vi "Go Home Sub_VI.vi"(8 "error in (no error)":errorcluster, 9 "stop":bool, 10 "Homing Freq":dbl format="%#_13g", 11 "Homing Duty %":dbl format="%#_13g") -> (0 "error out":errorcluster, 2 "Motor Status out":T2 {"Homing Duty %" format="%#_13g"; "Homing Freq" format="%#_13g"})   [LabVIEW 2017]
uses:
  X-Y Manipulator go home/Go Home State type def.ctl
panel:
  out "Y Velocity (mm/s)":dbl format="%#_3g"
  out "Y-axis distance":dbl
  out "X Velocity (mm/s)":dbl format="%#_3g"
  out "X-axis distance":dbl
  out "Y Axis State":T1
  out "X Axis state":T1
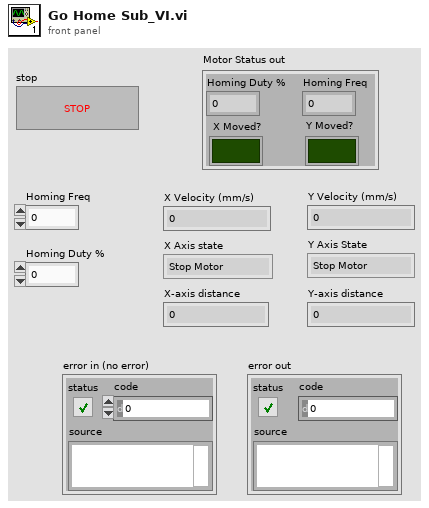
[diagram p1: front panel]
types:
  T1 = typedef "Go Home State type def.ctl" = enum16{"Stop Motor", "Read Input", "Drive Motor"}
  T2 = cluster{"Homing Freq":dbl, "Homing Duty %":dbl, "X Moved?":bool, "Y Moved?":bool}
  T3 = typedef "Encoder Count Direction Enum.ctl" = enum16{"Counting Up", "Counting Down"}
  T4 = cluster{"Y-axis rev count":dbl, "Y-axis distance":dbl, "X-axis rev count":dbl, "X-axis distance":dbl, "Y-axis direction":T3, "X-axis direction":T3, "X-counter val":i32, "Y-counter val":i32, "Reset X":bool, "Reset Y":bool}
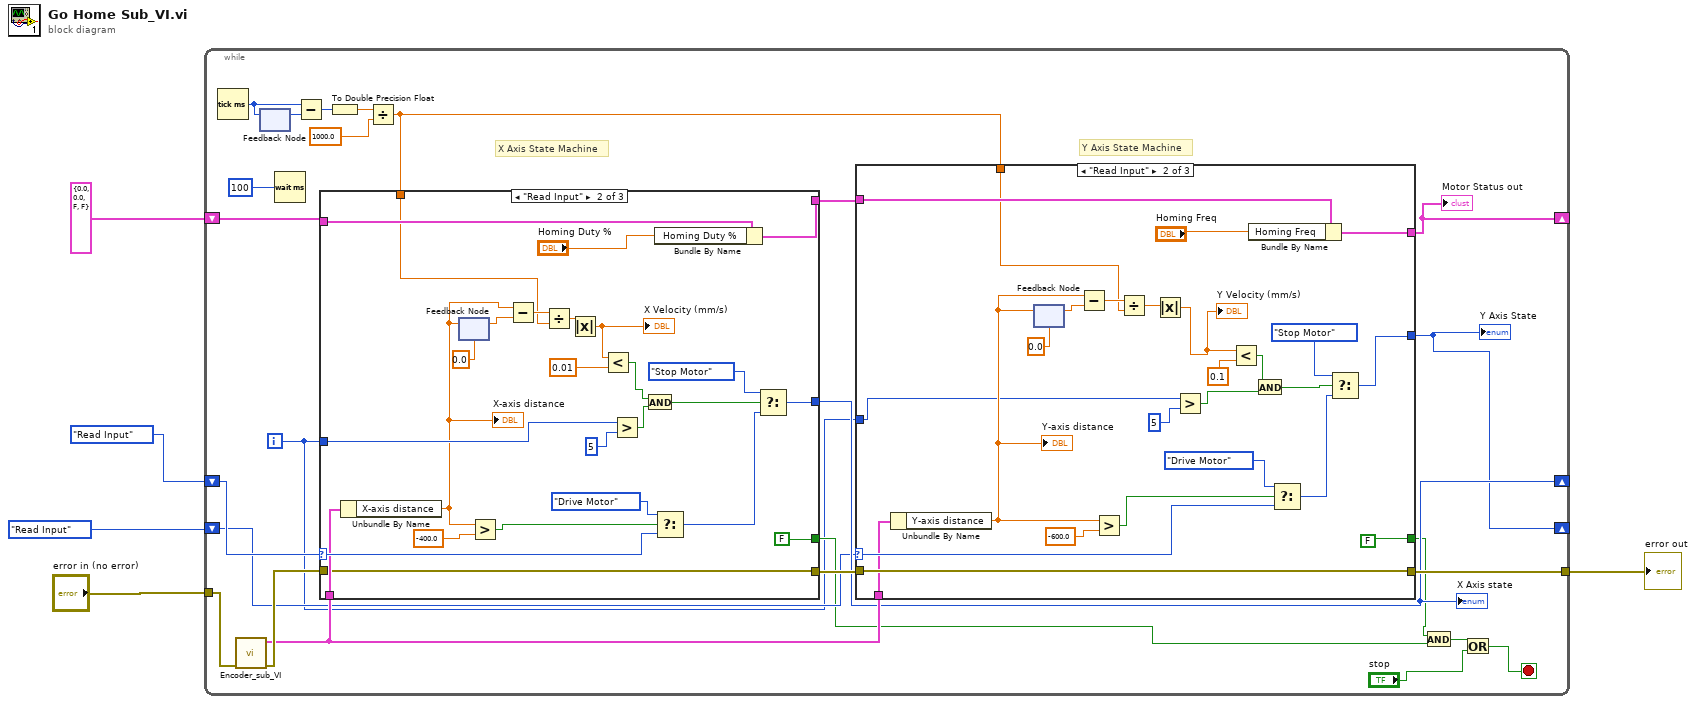
[diagram p0: block diagram]
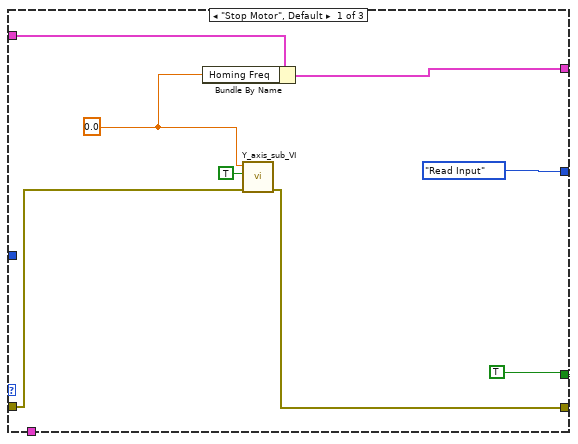
[diagram p2: hidden frame]
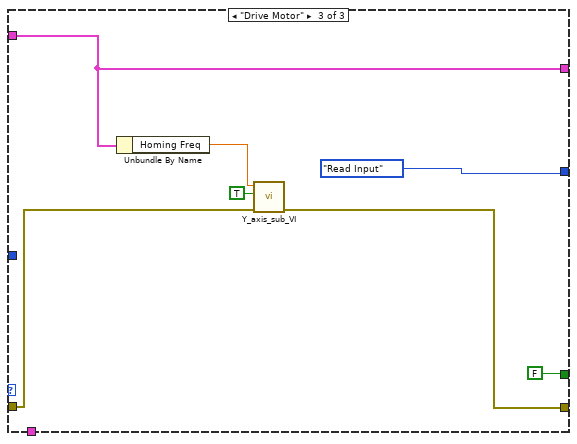
[diagram p3: hidden frame]
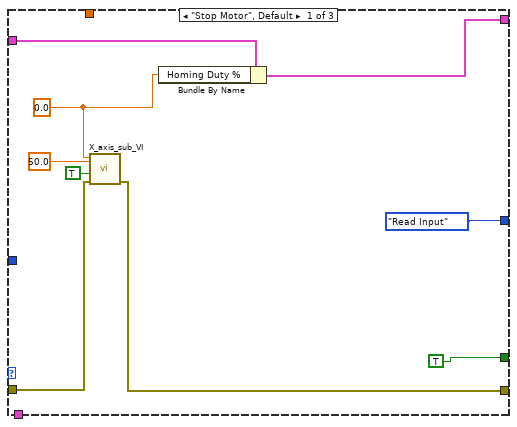
[diagram p4: hidden frame]
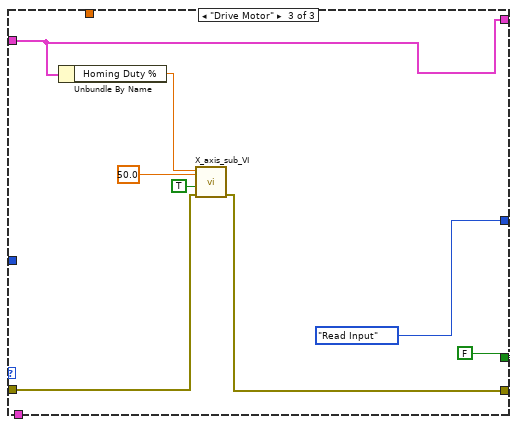
[diagram p5: hidden frame]
diagram:
  n1 = while {
    tunnel: "error in (no error)" -> [w29]
    tunnel: [w25] -> w2
    shift-right: [w21] -> _
    shift-left: Go_Home_State_type_def."Read Input" ("Enum 2") -> [w28]
    shift-right: [w26] -> _
    shift-left: T2 {"Homing Freq"=0.0, "Homing Duty %"=0.0, "X Moved?"=FALSE, "Y Moved?"=FALSE} ("Motor Status in") -> [w30]
    shift-right: [w20] -> _
    shift-left: Go_Home_State_type_def."Read Input" ("Enum") -> [w19]
    i -> [w6]
    stop <- w7 stop-if-true
    # "Y Axis State Machine"
    # "X Axis State Machine"
    n2 = Tick Count (ms)() -> (millisecond timer value=w15:u32)
    n3 = call "Encoder_sub_VI.vi"("error in (no error)"=w29) -> ("error out"=w23:errorcluster, "Encoder Output"=w22:T4)  [unwired: 9 in]
    n4 = feedback-in #1(w15) -> ()
    n5 = feedback #1() -> (w14:u32)  [unwired: 1 in]
    n6 = Wait (ms)(milliseconds to wait=u32 100) -> ()  [unwired: 1 out]
    n7 = Subtract(x=w15, y=w14) -> (x-y=w13:u32)
    n8 = To Double Precision Float(number=w13) -> (double precision float=w12:dbl)
    n9 = Divide(x=w12, y=1000.0) -> (x/y=w16:dbl)
    n10 = case shown="\"Read Input\"" w28 {
      selector: w28 -> [_ w103 _]
      tunnel: w30 -> [w80 w98 w107]
      tunnel: [w79 w105 w107] -> w27
      tunnel: [Go_Home_State_type_def."Read Input" w99 Go_Home_State_type_def."Read Input"] -> w21
      tunnel: w23 -> [w78 w93 w112]
      tunnel: [w73 w93 w111] -> w24
      tunnel: [TRUE FALSE FALSE] -> w10
      tunnel: w22 -> [_ w101 _]
      tunnel: w16 -> [_ w83 _]
      tunnel: w6 -> [_ w92 _]
      frame "Stop Motor", Default {
        w77 = 0.0
        n11 = call "X_axis_sub_VI.vi"("error in (no error)"=w78, "FWD/RVS"=TRUE, "Frequency"=50.0, "Duty Cycle %"=w77) -> ("error out"=w73:errorcluster)  [unwired: 7 in]
        n12 = Bundle By Name(cluster=w80, "Homing Duty %"=w77) -> (w79:T2)
      }
      frame "Read Input" {
        n13 = Unbundle By Name(w101) -> ("X-axis distance"=w87:dbl)
        "X-axis distance" <- w87
        n14 = feedback #2(0.0 ("X-axis distance")) -> (w86:dbl)
        n15 = feedback-in #2(w87) -> ()
        n16 = Greater?(x=w87, y=-400.0) -> (0:w97:bool)
        n17 = Subtract(x=w87, y=w86) -> (x-y=w84:dbl)
        n18 = Divide(x=w84, y=w83) -> (x/y=w82:dbl)
        n19 = Absolute Value(x=w82) -> (abs(x)=w81:dbl)
        "X Velocity (mm/s)" <- w81
        n20 = Less?(x=w81, y=0.01) -> (x < y?=w89:bool)
        n21 = Greater?(x=w92, y=5) -> (0:w90:bool)
        n22 = And(x=w89, y=w90) -> (x .and. y?=w88:bool)
        n23 = Bundle By Name(cluster=w98, "Homing Duty %"="Homing Duty %") -> (w105:T2)
        n24 = Select(t=Go_Home_State_type_def."Drive Motor", s=w97, f=w103) -> (s? t:f=w96:T1)
        n25 = Select(t=Go_Home_State_type_def."Stop Motor", s=w88, f=w96) -> (s? t:f=w99:T1)
      }
      frame "Drive Motor" {
        n26 = Unbundle By Name(w107) -> ("Homing Duty %"=w110:dbl)
        n27 = call "X_axis_sub_VI.vi"("error in (no error)"=w112, "FWD/RVS"=TRUE, "Frequency"=50.0, "Duty Cycle %"=w110) -> ("error out"=w111:errorcluster)  [unwired: 7 in]
      }
    }
    "X Axis state" <- w21
    n28 = case shown="\"Read Input\"" w19 {
      selector: w19 -> [_ w62 _]
      tunnel: [w38 w64 w65] -> w26
      tunnel: [Go_Home_State_type_def."Read Input" w60 Go_Home_State_type_def."Read Input"] -> w20
      tunnel: w24 -> [w31 w57 w69]
      tunnel: [w37 w57 w68] -> w25
      tunnel: [TRUE FALSE FALSE ("stop")] -> w11
      tunnel: w27 -> [w32 w55 w65]
      tunnel: w22 -> [_ w56 _]
      tunnel: w16 -> [_ w44 _]
      tunnel: w6 -> [_ w39 _]
      frame "Stop Motor", Default {
        w36 = 0.0
        n29 = Bundle By Name(cluster=w32, "Homing Freq"=w36) -> (w38:T2)
        n30 = call "Y_axis_sub_VI.vi"("error in (no error)"=w31, "FWD/RVS"=TRUE, "Frequency"=w36) -> ("error out"=w37:errorcluster)  [unwired: 8 in]
      }
      frame "Read Input" {
        n31 = Unbundle By Name(w56) -> ("Y-axis distance"=w43:dbl)
        "Y-axis distance" <- w43
        n32 = feedback #3(0.0 ("X-axis distance")) -> (w46:dbl)
        n33 = feedback-in #3(w43) -> ()
        n34 = Subtract(x=w43, y=w46) -> (x-y=w47:dbl)
        n35 = Greater?(x=w43, y=-600.0) -> (0:w53:bool)
        n36 = Divide(x=w47, y=w44) -> (x/y=w48:dbl)
        n37 = Absolute Value(x=w48) -> (abs(x)=w45:dbl)
        "Y Velocity (mm/s)" <- w45
        n38 = Greater?(x=w39, y=5) -> (0:w40:bool)
        n39 = Less?(x=w45, y=0.1) -> (x < y?=w50:bool)
        n40 = Bundle By Name(cluster=w55, "Homing Freq"="Homing Freq") -> (w64:T2)
        n41 = And(x=w50, y=w40) -> (x .and. y?=w51:bool)
        n42 = Select(t=Go_Home_State_type_def."Drive Motor", s=w53, f=w62) -> (s? t:f=w54:T1)
        n43 = Select(t=Go_Home_State_type_def."Stop Motor", s=w51, f=w54) -> (s? t:f=w60:T1)
      }
      frame "Drive Motor" {
        n44 = Unbundle By Name(w65) -> ("Homing Freq"=w66:dbl)
        n45 = call "Y_axis_sub_VI.vi"("error in (no error)"=w69, "FWD/RVS"=TRUE, "Frequency"=w66) -> ("error out"=w68:errorcluster)  [unwired: 8 in]
      }
    }
    "Motor Status out" <- w26
    "Y Axis State" <- w20
    n46 = And(x=w11, y=w10) -> (x .and. y?=w9:bool)
    n47 = Or(x=w9, y="stop") -> (x .or. y?=w7:bool)
  }
  "error out" <- w2
